vi "RTS Door Op Pattern.vi"(8 "Error In":errorcluster, 11 "Door Op Data Input":string[][](array[string])) -> (0 "Error Out":errorcluster, 3 "Door Op Pattern":T1[](array[typedef]))   [LabVIEW 2016]
uses:
  Type Definitions/RTS Door Open Close Pattern.ctl
  Type Definitions/RTS Door Action.ctl
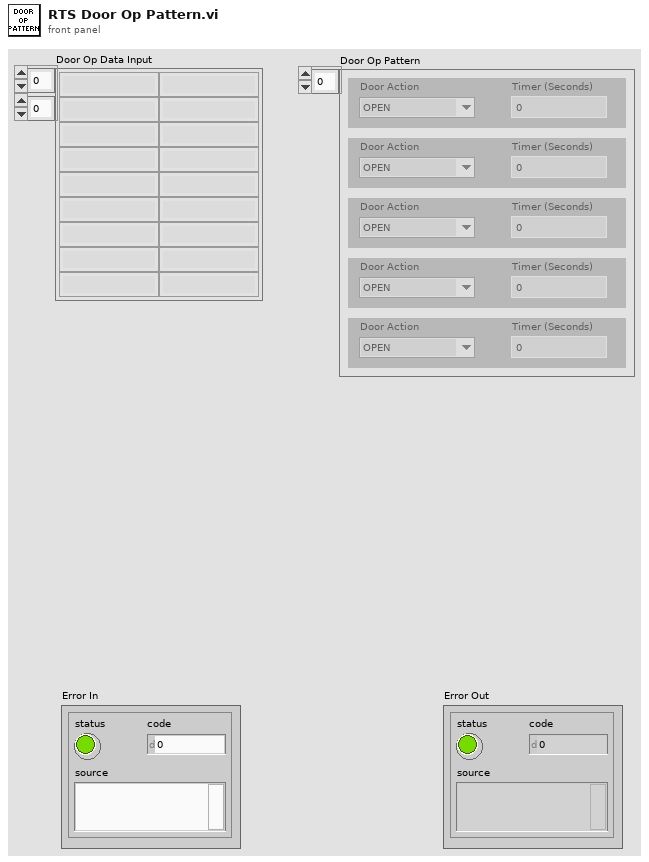
[diagram p1: front panel]
types:
  T1 = typedef "RTS Door Open Close Pattern.ctl" = cluster{"Door Action":T2, "Timer (Seconds)":u16}
  T2 = typedef "RTS Door Action.ctl" = enum16{"OPEN", "CLOSE", "DELAY", "REPEAT"}
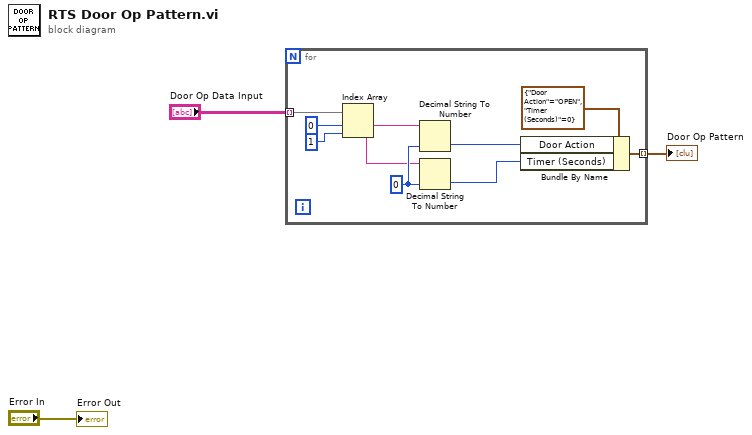
[diagram p0: block diagram]
diagram:
  n1 = for {
    tunnel: "Door Op Data Input" -> [w13] mode=indexing
    tunnel: [w5] -> w1 mode=indexing
    w9 = u16 0 ("default (0 I32)")
    n2 = Index Array(array=w13, index #1=0 ("index"), index #2=1 ("index")) -> (element #1=w10:string, element #2=w8:string)
    n3 = Decimal String To Number(string=w10, default (0L)=w9) -> (number=w7:u16)  [unwired: 1 in, 1 out]
    n4 = Decimal String To Number(string=w8, default (0L)=w9) -> (number=w6:u16)  [unwired: 1 in, 1 out]
    n5 = Bundle By Name(cluster=T1 {"Door Action"=enum."OPEN", "Timer (Seconds)"=0} ("Door Open/Close Pattern"), "Door Action"=w7, "Timer (Seconds)"=w6) -> (w5:T1)
  }
  "Door Op Pattern" <- w1
  "Error Out" <- "Error In"
